vi "Prepare for Close.vi"(8 "error in (no error)":errorcluster, 11 "Application Data in":T1) -> (0 "error out":errorcluster, 3 "Application Data out":T1)   [LabVIEW 2017, in "DSF Mini Explorer.lvlib"]
uses:
  DSF Configuration.llb/DSF Mini Explorer.lvlib
  Application Data.ctl
  Windows/DSF Core.lvlibp/Classes/Configuration/Configuration Session.lvclass
  View Mode.ctl
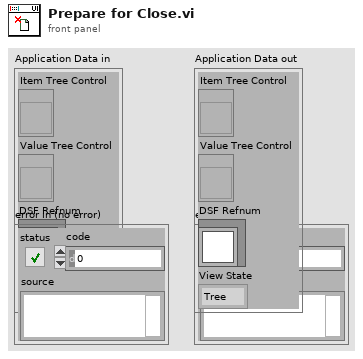
[diagram p1: front panel]
types:
  T1 = typedef "DSF Mini Explorer.lvlib/Application Data.ctl" = cluster{"Item Tree Control":refnum<vi>, "Value Tree Control":refnum<vi>, "DSF Refnum":refnum<class "Configuration Session.lvclass">, "View State":T2}
  T2 = typedef "DSF Mini Explorer.lvlib/View Mode.ctl" = enum16{"Tree", "List"}
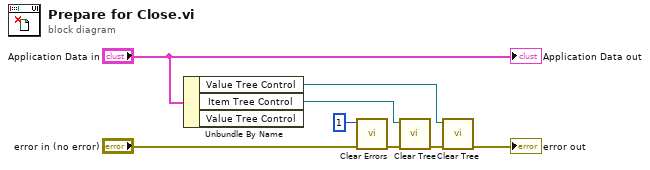
[diagram p0: block diagram]
diagram:
  n1 = Unbundle By Name("Application Data in") -> ("Value Tree Control"=w1:refnum<vi>, "Item Tree Control"=w3:refnum<vi>)  [unwired: 1 out]
  n2 = call "Clear Errors.vi"("error in (no error)"="error in (no error)", "specific error code to clear (0: all)"=1) -> ("error out"=w5:errorcluster)  [unwired: 4 in, 1 out]
  n3 = call "Clear Tree.vi"("error in (no error)"=w5, "TreeControl in"=w3) -> ("error out"=w4:errorcluster)  [unwired: 9 in]
  n4 = call "Clear Tree.vi"("error in (no error)"=w4, "TreeControl in"=w1) -> ("error out"=→"error out":errorcluster)  [unwired: 9 in]
  "Application Data out" <- "Application Data in"
